vi "Validate Response.vi"(11 "Port":i32) -> (0 "Error":errorcluster, 3 "Port":i32)   [LabVIEW 2010]
uses:
  Protocol Commands.ctl
  Command Classes.ctl
  LvSerial/LvSerial.llb/LvSerial.lvlib
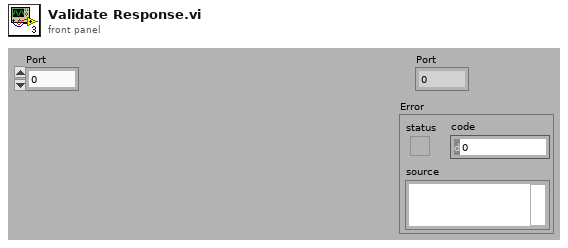
[diagram p1: front panel]
types:
  T1 = typedef "Command Classes.ctl" = enum8{"User Led", "Protocol", "MotorDriver"}
  T2 = typedef "Protocol Commands.ctl" = enum16{"Bad CRC", "Acknowledge", "Negative Acknowledge"}
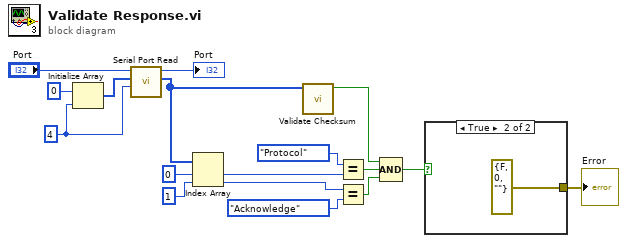
[diagram p0: block diagram]
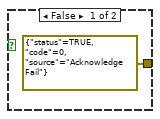
[diagram p2: hidden frame]
diagram:
  w15 = 4 ("Length")
  n1 = Initialize Array(u8 0 ("Length"), w15) -> (w16:u8[])
  n2 = call "Serial Port Read.vi"("Length"=w15, "Buffer"=w16, "Port"="Port") -> ("Buffer"=w3:u8[], "Port"=→"Port":i32)  [unwired: 7 in]
  n3 = Index Array(array=w3, index #1=0 ("index"), index #2=1 ("index")) -> (element #1=w13:u8, element #2=w11:u8)
  n4 = call "Validate Checksum.vi"("Buffer"=w3) -> ("Checksum Valid?"=w8:bool)  [unwired: 10 in]
  n5 = Equal?(x=Command_Classes."Protocol" ("Command Class"), y=w13) -> (x = y?=w9:bool)
  n6 = Equal?(x=w11, y=Protocol_Commands."Acknowledge" ("Protocol Commands")) -> (x = y?=w10:bool)
  n7 = Compound Arithmetic op=AND(w8, w9, w10) -> (w6:bool)
  n8 = case shown="True" w6 {
    tunnel: [errorcluster {"status"=TRUE, "code"=0, "source"="Acknowledge Fail"} ("error in (no error)") errorcluster {"status"=FALSE, "code"=0, "source"=""} ("error in (no error)")] -> w7
    frame False {
    }
    frame True {
    }
  }
  "Error" <- w7
